vi "File RIO_Get or Create Team Folder.vi"() -> (2 "error out":errorcluster, 3 "Team Files Folder":path)   [LabVIEW 2020]
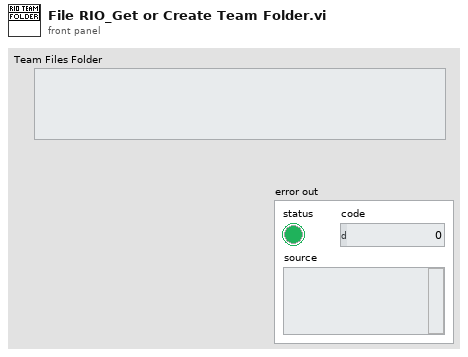
[diagram p1: front panel]
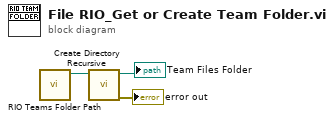
[diagram p0: block diagram]
diagram:
  n1 = call "RIO Teams Folder Path.vi"() -> ("Teams Folder"=w1:path)  [unwired: 10 in, 1 out]
  n2 = call <vilib>:"Create Directory Recursive.vi"("directory"=w1) -> ("error out"=→"error out":errorcluster, "directory copy"=→"Team Files Folder":path)  [unwired: 4 in, 1 out]
